vi "Scan tag to value.vi"(8 "error in (no error)":errorcluster, 10 "Index":i32, 11 "Data Type":T1) -> (0 "error out":errorcluster, 3 "Value":string)   [LabVIEW 2016, in "CVT.lvlib" / "Current Value Table.lvlib"]
uses:
  <vilib>/NI/Current Value Table/Current Value Table.lvlib
  <vilib>/NI/Current Value Table/Type Defs/Data Types.ctl
  <vilib>/NI/Current Value Table/DataTypes/Double_Data To ASCII String.vi
  <vilib>/NI/Current Value Table/DataTypes/Double_Read Index.vi
  <vilib>/NI/Current Value Table/DataTypes/Array of String_Data To ASCII String.vi
  <vilib>/NI/Current Value Table/DataTypes/Array of String_Read Index.vi
  <vilib>/NI/Current Value Table/DataTypes/Array of Boolean_Data To ASCII String.vi
  <vilib>/NI/Current Value Table/DataTypes/Array of Boolean_Read Index.vi
  <vilib>/NI/Current Value Table/DataTypes/Array of Single_Data To ASCII String.vi
  <vilib>/NI/Current Value Table/DataTypes/Array of Single_Read Index.vi
  <vilib>/NI/Current Value Table/DataTypes/Array of Double_Data To ASCII String.vi
  <vilib>/NI/Current Value Table/DataTypes/Array of Double_Read Index.vi
  <vilib>/NI/Current Value Table/DataTypes/Array of I8_Data To ASCII String.vi
  <vilib>/NI/Current Value Table/DataTypes/Array of I8_Read Index.vi
  <vilib>/NI/Current Value Table/DataTypes/Array of I16_Data To ASCII String.vi
  <vilib>/NI/Current Value Table/DataTypes/Array of I16_Read Index.vi
  <vilib>/NI/Current Value Table/DataTypes/Array of I32_Data To ASCII String.vi
  <vilib>/NI/Current Value Table/DataTypes/Array of I32_Read Index.vi
  <vilib>/NI/Current Value Table/DataTypes/Array of I64_Data To ASCII String.vi
  <vilib>/NI/Current Value Table/DataTypes/Array of I64_Read Index.vi
  <vilib>/NI/Current Value Table/DataTypes/Array of U64_Data To ASCII String.vi
  <vilib>/NI/Current Value Table/DataTypes/Array of U64_Read Index.vi
  <vilib>/NI/Current Value Table/DataTypes/Array of U32_Data To ASCII String.vi
  <vilib>/NI/Current Value Table/DataTypes/Array of U32_Read Index.vi
  <vilib>/NI/Current Value Table/DataTypes/Array of U16_Data To ASCII String.vi
  <vilib>/NI/Current Value Table/DataTypes/Array of U16_Read Index.vi
  <vilib>/NI/Current Value Table/DataTypes/Array of U8_Data To ASCII String.vi
  <vilib>/NI/Current Value Table/DataTypes/Array of U8_Read Index.vi
  <vilib>/NI/Current Value Table/DataTypes/Boolean_Data To ASCII String.vi
  <vilib>/NI/Current Value Table/DataTypes/Boolean_Read Index.vi
  <vilib>/NI/Current Value Table/DataTypes/String_Data To ASCII String.vi
  <vilib>/NI/Current Value Table/DataTypes/String_Read Index.vi
  <vilib>/NI/Current Value Table/DataTypes/U8_Data To ASCII String.vi
  <vilib>/NI/Current Value Table/DataTypes/U8_Read Index.vi
  <vilib>/NI/Current Value Table/DataTypes/U16_Data To ASCII String.vi
  <vilib>/NI/Current Value Table/DataTypes/U16_Read Index.vi
  <vilib>/NI/Current Value Table/DataTypes/U32_Data To ASCII String.vi
  <vilib>/NI/Current Value Table/DataTypes/U32_Read Index.vi
  <vilib>/NI/Current Value Table/DataTypes/U64_Data To ASCII String.vi
  <vilib>/NI/Current Value Table/DataTypes/U64_Read Index.vi
  <vilib>/NI/Current Value Table/DataTypes/I8_Data To ASCII String.vi
  <vilib>/NI/Current Value Table/DataTypes/I8_Read Index.vi
  <vilib>/NI/Current Value Table/DataTypes/I16_Data To ASCII String.vi
  <vilib>/NI/Current Value Table/DataTypes/I16_Read Index.vi
  <vilib>/NI/Current Value Table/DataTypes/I32_Data To ASCII String.vi
  <vilib>/NI/Current Value Table/DataTypes/I32_Read Index.vi
  <vilib>/NI/Current Value Table/DataTypes/I64_Data To ASCII String.vi
  <vilib>/NI/Current Value Table/DataTypes/I64_Read Index.vi
  <vilib>/NI/Current Value Table/DataTypes/Single_Data To ASCII String.vi
  <vilib>/NI/Current Value Table/DataTypes/Single_Read Index.vi
  <vilib>/NI/Current Value Table/Memory Block.vi
  <vilib>/NI/Current Value Table/DataTypes/Single_Memory Block.vi
  <vilib>/NI/Current Value Table/DataTypes/I64_Memory Block.vi
  <vilib>/NI/Current Value Table/DataTypes/I32_Memory Block.vi
  <vilib>/NI/Current Value Table/DataTypes/I16_Memory Block.vi
  <vilib>/NI/Current Value Table/DataTypes/I8_Memory Block.vi
  <vilib>/NI/Current Value Table/DataTypes/U64_Memory Block.vi
  <vilib>/NI/Current Value Table/DataTypes/U32_Memory Block.vi
  <vilib>/NI/Current Value Table/DataTypes/U16_Memory Block.vi
  <vilib>/NI/Current Value Table/DataTypes/U8_Memory Block.vi
  <vilib>/NI/Current Value Table/DataTypes/String_Memory Block.vi
  <vilib>/NI/Current Value Table/DataTypes/Boolean_Memory Block.vi
  <vilib>/NI/Current Value Table/DataTypes/Array of U8_Memory Block.vi
  <vilib>/NI/Current Value Table/DataTypes/Array of U16_Memory Block.vi
  <vilib>/NI/Current Value Table/DataTypes/Array of U32_Memory Block.vi
  <vilib>/NI/Current Value Table/DataTypes/Array of U64_Memory Block.vi
  <vilib>/NI/Current Value Table/DataTypes/Array of I64_Memory Block.vi
  <vilib>/NI/Current Value Table/DataTypes/Array of I32_Memory Block.vi
  <vilib>/NI/Current Value Table/DataTypes/Array of I16_Memory Block.vi
  <vilib>/NI/Current Value Table/DataTypes/Array of I8_Memory Block.vi
  <vilib>/NI/Current Value Table/DataTypes/Array of Double_Memory Block.vi
  <vilib>/NI/Current Value Table/DataTypes/Array of Single_Memory Block.vi
  <vilib>/NI/Current Value Table/DataTypes/Array of Boolean_Memory Block.vi
  <vilib>/NI/Current Value Table/DataTypes/Array of String_Memory Block.vi
  <vilib>/NI/Current Value Table/DataTypes/Double_Memory Block.vi
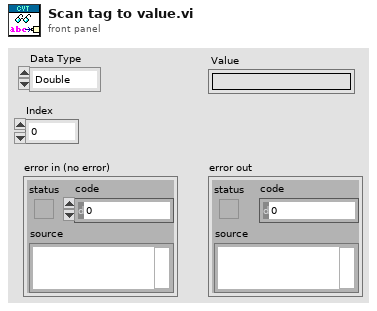
[diagram p1: front panel]
types:
  T1 = typedef "CVT.lvlib/Current Value Table.lvlib/Data Types.ctl" = enum16{"Double", "Single", "I64", "I32", "I16", "I8", "U64", "U32", "U16", "U8", "String", "Boolean", "Array of U8", "Array of U16", "Array of U32", "Array of U64", "Array of I64", "Array of I32", "Array of I16", "Array of I8", "Array of Double", "Array of Single", "Array of Boolean", "Array of String"}
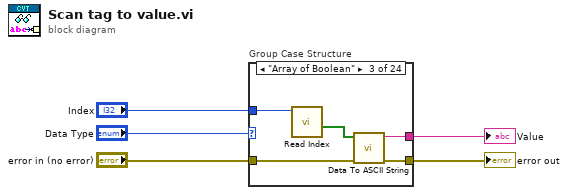
[diagram p0: block diagram]
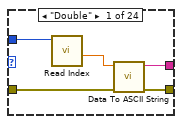
[diagram p2: hidden frame]
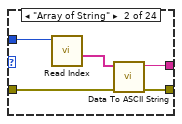
[diagram p3: hidden frame]
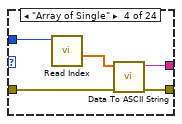
[diagram p4: hidden frame]
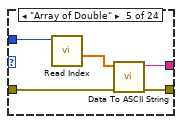
[diagram p5: hidden frame]
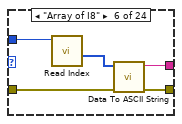
[diagram p6: hidden frame]
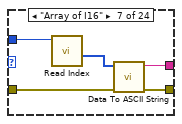
[diagram p7: hidden frame]
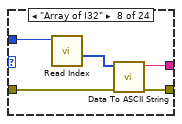
[diagram p8: hidden frame]
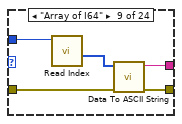
[diagram p9: hidden frame]
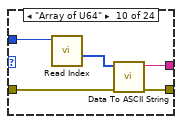
[diagram p10: hidden frame]
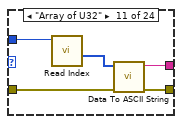
[diagram p11: hidden frame]
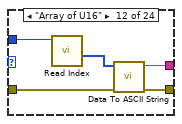
[diagram p12: hidden frame]
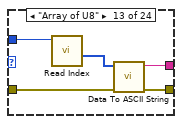
[diagram p13: hidden frame]
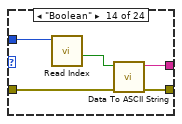
[diagram p14: hidden frame]
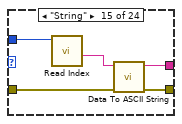
[diagram p15: hidden frame]
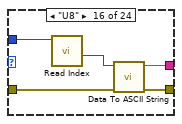
[diagram p16: hidden frame]
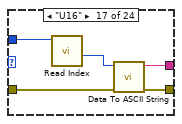
[diagram p17: hidden frame]
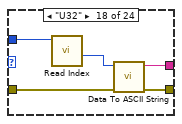
[diagram p18: hidden frame]
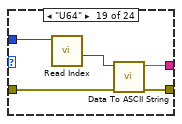
[diagram p19: hidden frame]
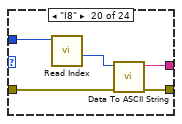
[diagram p20: hidden frame]
diagram:
  n1 = case "Group Case Structure" shown="\"Array of Boolean\"" "Data Type" {
    tunnel: "error in (no error)" -> [w7 w12 w17 w22 w27 w32 w37 w42 w47 w52 w57 w62 w67 w72 w77 w82 w87 w92 w97 w102 w107 w112 w117 w122]
    tunnel: [w10 w15 w20 w25 w30 w35 w40 w45 w50 w55 w60 w65 w70 w75 w80 w85 w90 w95 w100 w105 w110 w115 w120 w125] -> w1
    tunnel: [w9 w14 w19 w24 w29 w34 w39 w44 w49 w54 w59 w64 w69 w74 w79 w84 w89 w94 w99 w104 w109 w114 w119 w124] -> w2
    tunnel: "Index" -> [w6 w11 w16 w21 w26 w31 w36 w41 w46 w51 w56 w61 w66 w71 w76 w81 w86 w91 w96 w101 w106 w111 w116 w121]
    frame "Double" {
      n2 = call-poly <vilib>:"Read Index.vi"("Index"=w6) -> ("Value"=w8:dbl)  [unwired: 10 in]
      n3 = call-poly <vilib>:"Data To ASCII String.vi"("error in"=w7, "Data"=w8) -> ("error out"=w10:errorcluster, "Value"=w9:string)  [unwired: 8 in]
    }
    frame "Array of String" {
      n4 = call-poly <vilib>:"Read Index.vi"("Index"=w11) -> ("Value"=w13:string[])  [unwired: 10 in]
      n5 = call-poly <vilib>:"Data To ASCII String.vi"("error in"=w12, "Data"=w13) -> ("error out"=w15:errorcluster, "Value"=w14:string)  [unwired: 8 in]
    }
    frame "Array of Boolean" {
      n6 = call-poly <vilib>:"Read Index.vi"("Index"=w16) -> ("Value"=w18:bool[])  [unwired: 10 in]
      n7 = call-poly <vilib>:"Data To ASCII String.vi"("error in"=w17, "Data"=w18) -> ("error out"=w20:errorcluster, "Value"=w19:string)  [unwired: 8 in]
    }
    frame "Array of Single" {
      n8 = call-poly <vilib>:"Read Index.vi"("Index"=w21) -> ("Value"=w23:sgl[])  [unwired: 10 in]
      n9 = call-poly <vilib>:"Data To ASCII String.vi"("error in"=w22, "Data"=w23) -> ("error out"=w25:errorcluster, "Value"=w24:string)  [unwired: 8 in]
    }
    frame "Array of Double" {
      n10 = call-poly <vilib>:"Read Index.vi"("Index"=w26) -> ("Value"=w28:dbl[])  [unwired: 10 in]
      n11 = call-poly <vilib>:"Data To ASCII String.vi"("error in"=w27, "Data"=w28) -> ("error out"=w30:errorcluster, "Value"=w29:string)  [unwired: 8 in]
    }
    frame "Array of I8" {
      n12 = call-poly <vilib>:"Read Index.vi"("Index"=w31) -> ("Value"=w33:i8[])  [unwired: 10 in]
      n13 = call-poly <vilib>:"Data To ASCII String.vi"("error in"=w32, "Data"=w33) -> ("error out"=w35:errorcluster, "Value"=w34:string)  [unwired: 8 in]
    }
    frame "Array of I16" {
      n14 = call-poly <vilib>:"Read Index.vi"("Index"=w36) -> ("Value"=w38:i16[])  [unwired: 10 in]
      n15 = call-poly <vilib>:"Data To ASCII String.vi"("error in"=w37, "Data"=w38) -> ("error out"=w40:errorcluster, "Value"=w39:string)  [unwired: 8 in]
    }
    frame "Array of I32" {
      n16 = call-poly <vilib>:"Read Index.vi"("Index"=w41) -> ("Value"=w43:i32[])  [unwired: 10 in]
      n17 = call-poly <vilib>:"Data To ASCII String.vi"("error in"=w42, "Data"=w43) -> ("error out"=w45:errorcluster, "Value"=w44:string)  [unwired: 8 in]
    }
    frame "Array of I64" {
      n18 = call-poly <vilib>:"Read Index.vi"("Index"=w46) -> ("Value"=w48:i64[])  [unwired: 10 in]
      n19 = call-poly <vilib>:"Data To ASCII String.vi"("error in"=w47, "Data"=w48) -> ("error out"=w50:errorcluster, "Value"=w49:string)  [unwired: 8 in]
    }
    frame "Array of U64" {
      n20 = call-poly <vilib>:"Read Index.vi"("Index"=w51) -> ("Value"=w53:u64[])  [unwired: 10 in]
      n21 = call-poly <vilib>:"Data To ASCII String.vi"("error in"=w52, "Data"=w53) -> ("error out"=w55:errorcluster, "Value"=w54:string)  [unwired: 8 in]
    }
    frame "Array of U32" {
      n22 = call-poly <vilib>:"Read Index.vi"("Index"=w56) -> ("Value"=w58:u32[])  [unwired: 10 in]
      n23 = call-poly <vilib>:"Data To ASCII String.vi"("error in"=w57, "Data"=w58) -> ("error out"=w60:errorcluster, "Value"=w59:string)  [unwired: 8 in]
    }
    frame "Array of U16" {
      n24 = call-poly <vilib>:"Read Index.vi"("Index"=w61) -> ("Value"=w63:u16[])  [unwired: 10 in]
      n25 = call-poly <vilib>:"Data To ASCII String.vi"("error in"=w62, "Data"=w63) -> ("error out"=w65:errorcluster, "Value"=w64:string)  [unwired: 8 in]
    }
    frame "Array of U8" {
      n26 = call-poly <vilib>:"Read Index.vi"("Index"=w66) -> ("Value"=w68:u8[])  [unwired: 10 in]
      n27 = call-poly <vilib>:"Data To ASCII String.vi"("error in"=w67, "Data"=w68) -> ("error out"=w70:errorcluster, "Value"=w69:string)  [unwired: 8 in]
    }
    frame "Boolean" {
      n28 = call-poly <vilib>:"Read Index.vi"("Index"=w71) -> ("Value"=w73:bool)  [unwired: 10 in]
      n29 = call-poly <vilib>:"Data To ASCII String.vi"("error in"=w72, "Data"=w73) -> ("error out"=w75:errorcluster, "Value"=w74:string)  [unwired: 8 in]
    }
    frame "String" {
      n30 = call-poly <vilib>:"Read Index.vi"("Index"=w76) -> ("Value"=w78:string)  [unwired: 10 in]
      n31 = call-poly <vilib>:"Data To ASCII String.vi"("error in"=w77, "Data"=w78) -> ("error out"=w80:errorcluster, "Value"=w79:string)  [unwired: 8 in]
    }
    frame "U8" {
      n32 = call-poly <vilib>:"Read Index.vi"("Index"=w81) -> ("Value"=w83:u8)  [unwired: 10 in]
      n33 = call-poly <vilib>:"Data To ASCII String.vi"("error in"=w82, "Data"=w83) -> ("error out"=w85:errorcluster, "Value"=w84:string)  [unwired: 8 in]
    }
    frame "U16" {
      n34 = call-poly <vilib>:"Read Index.vi"("Index"=w86) -> ("Value"=w88:u16)  [unwired: 10 in]
      n35 = call-poly <vilib>:"Data To ASCII String.vi"("error in"=w87, "Data"=w88) -> ("error out"=w90:errorcluster, "Value"=w89:string)  [unwired: 8 in]
    }
    frame "U32" {
      n36 = call-poly <vilib>:"Read Index.vi"("Index"=w91) -> ("Value"=w93:u32)  [unwired: 10 in]
      n37 = call-poly <vilib>:"Data To ASCII String.vi"("error in"=w92, "Data"=w93) -> ("error out"=w95:errorcluster, "Value"=w94:string)  [unwired: 8 in]
    }
    frame "U64" {
      n38 = call-poly <vilib>:"Read Index.vi"("Index"=w96) -> ("Value"=w98:u64)  [unwired: 10 in]
      n39 = call-poly <vilib>:"Data To ASCII String.vi"("error in"=w97, "Data"=w98) -> ("error out"=w100:errorcluster, "Value"=w99:string)  [unwired: 8 in]
    }
    frame "I8" {
      n40 = call-poly <vilib>:"Read Index.vi"("Index"=w101) -> ("Value"=w103:i8)  [unwired: 10 in]
      n41 = call-poly <vilib>:"Data To ASCII String.vi"("error in"=w102, "Data"=w103) -> ("error out"=w105:errorcluster, "Value"=w104:string)  [unwired: 8 in]
    }
    frame "I16" {
      n42 = call-poly <vilib>:"Read Index.vi"("Index"=w106) -> ("Value"=w108:i16)  [unwired: 10 in]
      n43 = call-poly <vilib>:"Data To ASCII String.vi"("error in"=w107, "Data"=w108) -> ("error out"=w110:errorcluster, "Value"=w109:string)  [unwired: 8 in]
    }
    frame "I32" {
      n44 = call-poly <vilib>:"Read Index.vi"("Index"=w111) -> ("Value"=w113:i32)  [unwired: 10 in]
      n45 = call-poly <vilib>:"Data To ASCII String.vi"("error in"=w112, "Data"=w113) -> ("error out"=w115:errorcluster, "Value"=w114:string)  [unwired: 8 in]
    }
    frame "I64" {
      n46 = call-poly <vilib>:"Read Index.vi"("Index"=w116) -> ("Value"=w118:i64)  [unwired: 10 in]
      n47 = call-poly <vilib>:"Data To ASCII String.vi"("error in"=w117, "Data"=w118) -> ("error out"=w120:errorcluster, "Value"=w119:string)  [unwired: 8 in]
    }
    frame "Single" {
      n48 = call-poly <vilib>:"Read Index.vi"("Index"=w121) -> ("Value"=w123:sgl)  [unwired: 10 in]
      n49 = call-poly <vilib>:"Data To ASCII String.vi"("error in"=w122, "Data"=w123) -> ("error out"=w125:errorcluster, "Value"=w124:string)  [unwired: 8 in]
    }
  }
  "Value" <- w2
  "error out" <- w1
